vi "Untitled 1.vi"() -> ()   [LabVIEW 2023]
uses:
  System.Drawing
  <vilib>/picture/picture.llb/Draw True-Color Pixmap.vi
  Glyph .NET Drawer/Drawer .Net.lvclass
panel:
  out "Numeric":i32
  in  "stop":bool
  in  "angle":sgl=3.0
  in  "Offset":cluster{"X":sgl, "Y":sgl}
  out "2D Picture":picture
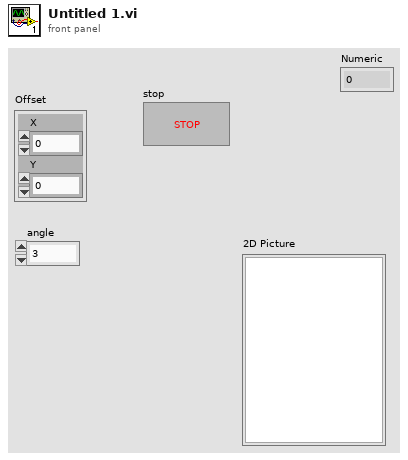
[diagram p1: front panel]
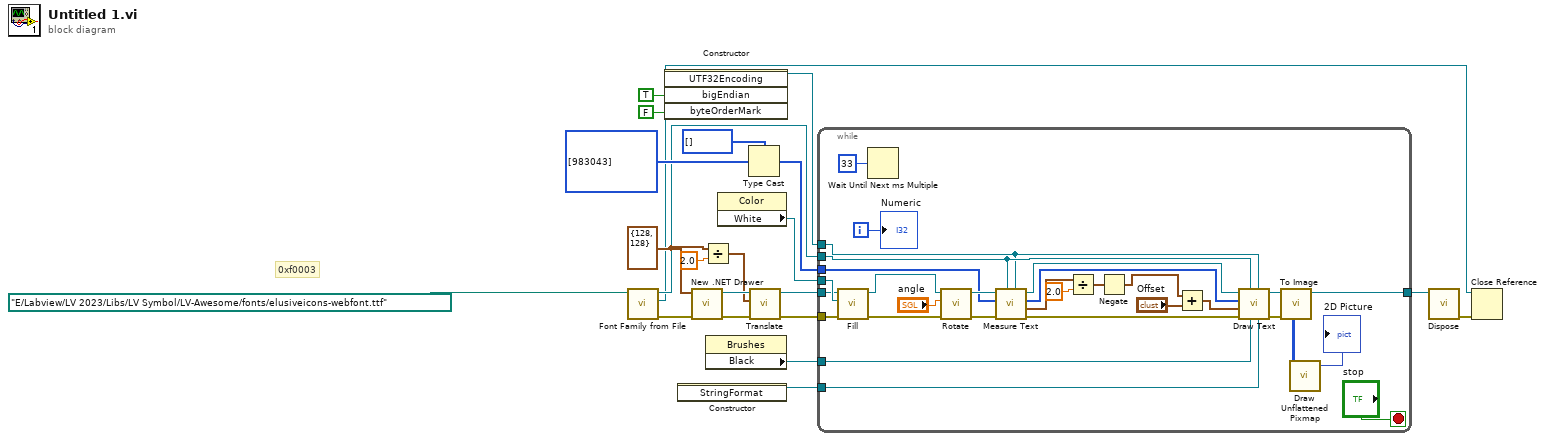
[diagram p0: block diagram]
diagram:
  w5 = cluster{"width":i32, "height":i32} {"width"=128, "height"=128} ("Size")
  # "0xf0003"
  n1 = call "Font Family from File.vi"("Path"=path "E:/Labview/LV 2023/Libs/LV Symbol/LV-Awesome/fonts/elusiveicons-webfont.ttf") -> ("error out"=w7:errorcluster, "FontCollection"=w2:refnum<k24>, "Font"=w6:refnum<k24>)  [unwired: 8 in]
  n2 = constructor class="UTF32Encoding"("bigEndian"=TRUE, "byteOrderMark"=FALSE) -> (reference out=w14:refnum<k24>)  [unwired: 3 in, 4 out]
  n3 = constructor class="StringFormat"() -> (reference out=w13:refnum<k24>)  [unwired: 3 in, 2 out]
  n4 = call "New .NET Drawer.vi"("error in (no error)"=w7, "Size"=w5) -> ("error out"=w8:errorcluster, "Canvas out"=w12:refnum<class "Drawer .Net.lvclass">)  [unwired: 8 in]
  n5 = Divide(x=w5, y=sgl 2.0) -> (x/y=w1:cluster{"width":sgl, "height":sgl})
  n6 = property class="Brushes"() -> ("Black"=w19:refnum<k24>)  [unwired: 2 in, 2 out]
  n7 = property class="Color"() -> ("White"=w21:refnum<k24>)  [unwired: 2 in, 2 out]
  n8 = Type Cast(type=u8[] [], x=u32[] [983043]) -> (*(type *) &x=w18:u8[])
  n9 = call "Translate.vi"("error in (no error)"=w8, "Offset"=w1, "Canvas in"=w12) -> ("error out"=w9:errorcluster, "Canvas out"=w11:refnum<class "Drawer .Net.lvclass">)  [unwired: 7 in]
  n10 = while {
    tunnel: w21 -> [w52]
    tunnel: w19 -> [w51]
    tunnel: w6 -> [w30]
    tunnel: w18 -> [w28]
    tunnel: w14 -> [w29]
    tunnel: w13 -> [w50]
    tunnel: w11 -> [w42]
    tunnel: [w39] -> w10
    tunnel: w9 -> [w38]
    i -> [w27]
    stop <- "stop" stop-if-true
    n11 = call "Fill.vi"("error in (no error)"=w38, "Color"=w52, "Canvas in"=w42) -> ("error out"=w37:errorcluster, "Canvas out"=w40:refnum<class "Drawer .Net.lvclass">)  [unwired: 7 in]
    n12 = Wait Until Next ms Multiple(millisecond multiple=33) -> ()  [unwired: 1 out]
    n13 = call "Rotate.vi"("error in (no error)"=w37, "angle"="angle", "Canvas in"=w40) -> ("error out"=w36:errorcluster, "Canvas out"=w35:refnum<class "Drawer .Net.lvclass">)  [unwired: 7 in]
    n14 = call "Measure Text.vi"("Encoding"=w29, "Font"=w30, "error in (no error)"=w36, "Text Raw"=w28, "Canvas in"=w35) -> ("error out"=w32:errorcluster, "Size"=w26:cluster{"Width":sgl, "Height":sgl}, "Text Raw"=w25:u8[], "Canvas out"=w34:refnum<class "Drawer .Net.lvclass">)  [unwired: 3 in]
    n15 = Divide(x=w26, y=sgl 2.0) -> (x/y=w46:cluster{"Width":sgl, "Height":sgl})
    n16 = Negate(x=w46) -> (-x=w44:cluster{"Width":sgl, "Height":sgl})
    n17 = Add(x=w44, y="Offset") -> (x+y=w43:cluster{sgl, sgl})
    n18 = call "Draw Text.vi"("Text Format"=w50, "Encoding"=w29, "Brush"=w51, "Font"=w30, "error in (no error)"=w32, "Offset"=w43, "Bytes"=w25, "Canvas in"=w34) -> ("error out"=w49:errorcluster, "Canvas out"=w33:refnum<class "Drawer .Net.lvclass">)  [unwired: 2 in]
    n19 = call "To Image.vi"("error in (no error)"=w49, "Canvas in"=w33) -> ("Bitmap"=w24:u32[][], "Canvas out"=w39:refnum<class "Drawer .Net.lvclass">)  [unwired: 7 in, 1 out]
    n20 = call-poly <vilib>:"Draw Unflattened Pixmap.vi"("data (RGB format)"=w24) -> ("new picture"=→"2D Picture":picture)  [unwired: 8 in]
    "Numeric" <- w27
  }
  n21 = call-dynamic "Dispose.vi"("Canvas in"=w10) -> ("error out"=w3:errorcluster)  [unwired: 10 in]
  n22 = Close Reference(reference=w2, error in (no error)=w3) -> ()  [unwired: 1 out]
